vi "(-1)^x.vi"(1 "x":i32) -> (0 "(-1)^x":i32)   [LabVIEW 2009]
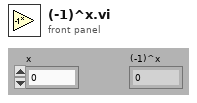
[diagram p1: front panel]
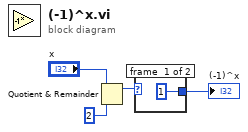
[diagram p0: block diagram]
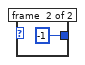
[diagram p2: hidden frame]
diagram:
  n1 = Quotient & Remainder(x="x", y=2) -> (x-y*floor(x/y)=w1:i32)  [unwired: 1 out]
  n2 = case shown="0, Default" w1 {
    tunnel: [1 -1] -> w4
    frame #0 {
    }
    frame #1 {
    }
  }
  "(-1)^x" <- w4
